vi "HFRR ADV v01.vi"() -> ()   [LabVIEW 2023] (continued)
        n1660 = property on="Language Selection" class="Enum (strict)"("Visible"=w1316) -> ()  [unwired: 2 in, 2 out]
        n1661 = property on="File Path" class="Path"("Disabled"=w1317) -> ()  [unwired: 2 in, 2 out]
        n1662 = property on="TEMP INTERCEPT:" class="DigNum (strict)"("Disabled"=w1317) -> ()  [unwired: 2 in, 2 out]
        n1663 = property on="visa due" class="CmbBox"("Disabled"=w1317) -> ()  [unwired: 2 in, 2 out]
        n1664 = property on="AIR TEMP INTERCEPT:" class="DigNum (strict)"("Disabled"=w1317) -> ()  [unwired: 2 in, 2 out]
        n1665 = property on="CH-HUMIDITY DRY" class="DigNum (strict)"("Disabled"=w1317) -> ()  [unwired: 2 in, 2 out]
        n1666 = property on="CH-HUMIDITY WET" class="DigNum (strict)"("Disabled"=w1317) -> ()  [unwired: 2 in, 2 out]
        n1667 = property on="CH-POWER -" class="DigNum (strict)"("Disabled"=w1317) -> ()  [unwired: 2 in, 2 out]
        n1668 = property on="CH-HEATER" class="DigNum (strict)"("Disabled"=w1317) -> ()  [unwired: 2 in, 2 out]
        n1669 = property on="CH-POWER +" class="DigNum (strict)"("Disabled"=w1317) -> ()  [unwired: 2 in, 2 out]
        n1670 = property on="SrvM CP" class="Bool (strict)"("Disabled"=w1317) -> ()  [unwired: 2 in, 2 out]
        n1671 = property on="Stroke PID Gains" class="Clust (strict)"("Disabled"=w1317) -> ()  [unwired: 2 in, 2 out]
        n1672 = property on="STROKE GAIN :" class="DigNum (strict)"("Disabled"=w1317) -> ()  [unwired: 2 in, 2 out]
        n1673 = property on="LvdtOff" class="DigNum (strict)"("Disabled"=w1317) -> ()  [unwired: 2 in, 2 out]
        n1674 = property on="DISPLACEMENT :" class="DigNum (strict)"("Disabled"=w1317) -> ()  [unwired: 2 in, 2 out]
        n1675 = property on="Port 2 Error" class="Clust (strict)"("Visible"="EDIT") -> ()  [unwired: 2 in, 2 out]
        n1676 = property on="Port 1 Error" class="Clust (strict)"("Visible"="EDIT") -> ()  [unwired: 2 in, 2 out]
        n1677 = stacked-sequence {
          frame #0 {
            n1678 = local read "EDIT"() -> (w1368:bool)
            n1679 = case shown="False" w1368 {
              tunnel: [u8 2 ("Disabled") u8 0 ("Disabled")] -> _
              frame False {
                w1370 = FALSE
                n1680 = local write "Password"("") -> ()
                n1681 = property on="ENTER THE NEW PASSWORD" class="Str"("Visible"=w1370) -> ()  [unwired: 2 in, 2 out]
                n1682 = property on="ENTER CURRENT PASSWORD" class="Str"("Visible"=w1370) -> ()  [unwired: 2 in, 2 out]
                n1683 = property on="SrvM CP" class="Bool (strict)"("Visible"=w1370) -> ()  [unwired: 2 in, 2 out]
                n1684 = property on="Password" class="Str"("Visible"=w1370) -> ()  [unwired: 2 in, 2 out]
                n1685 = local write "x = y?"(w1370) -> ()
                n1686 = local write "SrvM CP"(w1370) -> ()
                n1687 = property on="message" class="Str"("Visible"=w1370) -> ()  [unwired: 2 in, 2 out]
              }
              frame True {
                w1373 = TRUE
                n1688 = property on="SrvM CP" class="Bool (strict)"("Visible"=w1373) -> ()  [unwired: 2 in, 2 out]
                n1689 = property on="Password" class="Str"("Visible"=w1373) -> ()  [unwired: 2 in, 2 out]
              }
            }
            "dipl pwd" <- "@143$\n" ("dipl pwd")
          }
          frame #1 {
            # "Gain password"
            n1690 = String To Byte Array(string="ENTER CURRENT PASSWORD") -> (unsigned byte array=w1378:u8[])
            n1691 = Search 1D Array(1D array=w1378, element=u8 10) -> (index of element=w1381:i32)  [unwired: 1 in]
            n1692 = Index Array(array=w1378, index=w1381) -> (element=w1377:u8)
            n1693 = Equal?(x=w1377, y=10) -> (x = y?=w1375:bool)
            n1694 = case shown="True" w1375 {
              frame False {
                n1695 = property on="ENTER THE NEW PASSWORD" class="Str"("Visible"=FALSE) -> ()  [unwired: 2 in, 2 out]
              }
              frame True {
                # "password"
                # "change password logic"
                n1696 = local read "dipl pwd"() -> (w1388:string)
                n1697 = local read "ENTER CURRENT PASSWORD"() -> (w1394:string)
                n1698 = String To Byte Array(string=w1394) -> (unsigned byte array=w1396:u8[])
                n1699 = Array Size(array=w1396) -> (size(s)=w1393:i32)
                n1700 = String To Byte Array(string=w1388) -> (unsigned byte array=w1389:u8[])
                n1701 = Array Size(array=w1389) -> (size(s)=w1391:i32)
                n1702 = for {
                  N: w1393 -> [_]
                  tunnel: w1396 -> [w1420]
                  tunnel: [w1418] -> w1397 mode=indexing
                  tunnel: w1393 -> [w1412]
                  i -> [w1413]
                  n1703 = Decrement(x=w1412) -> (x-1=w1410:i32)
                  n1704 = Index Array(array=w1420, index=w1413) -> (element=w1414:u8)
                  n1705 = Equal?(x=w1413, y=w1410) -> (x = y?=w1411:bool)
                  n1706 = Number To Decimal String(number=w1414) -> (decimal integer string=w1419:string)  [unwired: 1 in]
                  n1707 = Select(t="", s=w1411, f="\r") -> (s? t:f=w1416:string)
                  n1708 = Concatenate Strings(w1419, w1416) -> (w1418:string)
                }
                n1709 = for {
                  N: w1391 -> [_]
                  tunnel: w1389 -> [w1408]
                  tunnel: [w1406] -> w1390 mode=indexing
                  tunnel: w1391 -> [w1403]
                  i -> [w1404]
                  n1710 = Decrement(x=w1403) -> (x-1=w1402:i32)
                  n1711 = Index Array(array=w1408, index=w1404) -> (element=w1407:u8)
                  n1712 = Equal?(x=w1404, y=w1402) -> (x = y?=w1401:bool)
                  n1713 = Number To Decimal String(number=w1407) -> (decimal integer string=w1405:string)  [unwired: 1 in]
                  n1714 = Select(t="", s=w1401, f="\r") -> (s? t:f=w1398:string)
                  n1715 = Concatenate Strings(w1405, w1398) -> (w1406:string)
                }
                n1716 = local read "string"() -> (w1395:string)
                n1717 = Concatenate Strings(w1397) -> (w1385:string)
                n1718 = Concatenate Strings(w1390) -> (w1384:string)
                n1719 = Concatenate Strings(w1395) -> (w1392:string)
                n1720 = Equal?(x=w1385, y=w1384) -> (x = y?=w1383:bool)
                n1721 = Equal?(x=w1385, y=w1392) -> (x = y?=w1387:bool)
                n1722 = Or(x=w1387, y=w1383) -> (x .or. y?=w1386:bool)
                n1723 = case shown="True" w1386 {
                  frame False {
                  }
                  frame True {
                    n1724 = property on="ENTER THE NEW PASSWORD" class="Str"("Visible"=TRUE) -> ()  [unwired: 2 in, 2 out]
                  }
                }
              }
            }
          }
          frame #2 {
            n1725 = String To Byte Array(string="ENTER THE NEW PASSWORD") -> (unsigned byte array=w1423:u8[])
            n1726 = Search 1D Array(1D array=w1423, element=u8 10) -> (index of element=w1427:i32)  [unwired: 1 in]
            n1727 = Index Array(array=w1423, index=w1427) -> (element=w1425:u8)
            n1728 = Equal?(x=w1425, y=10) -> (x = y?=w1422:bool)
            n1729 = case shown="True" w1422 {
              frame False {
              }
              frame True {
                n1730 = local read "ENTER THE NEW PASSWORD"() -> (w1430:string)
                n1731 = String To Byte Array(string=w1430) -> (unsigned byte array=w1435:u8[])
                n1732 = Array Size(array=w1435) -> (size(s)=w1432:i32)
                n1733 = for {
                  N: w1432 -> [_]
                  tunnel: w1435 -> [w1448]
                  tunnel: [w1445] -> w1437 mode=indexing
                  tunnel: w1432 -> [w1440]
                  i -> [w1438]
                  n1734 = Index Array(array=w1448, index=w1438) -> (element=w1447:u8)
                  n1735 = Decrement(x=w1440) -> (x-1=w1441:i32)
                  n1736 = Equal?(x=w1438, y=w1441) -> (x = y?=w1442:bool)
                  n1737 = Number To Decimal String(number=w1447) -> (decimal integer string=w1446:string)  [unwired: 1 in]
                  n1738 = Select(t="", s=w1442, f="\r") -> (s? t:f=w1439:string)
                  n1739 = Concatenate Strings(w1446, w1439) -> (w1445:string)
                }
                n1740 = local write "SrvM CP"(FALSE) -> ()
                n1741 = local write "EDIT"(FALSE) -> ()
                n1742 = local read "file path"() -> (w1429:path)
                n1743 = Concatenate Strings(w1437) -> (w1431:string)
                n1744 = Delete(path (use dialog)=w1429) -> (deleted path=w1433:path)  [unwired: 4 in, 2 out]
                n1745 = call <vilib>:"Write Characters To File.vi"("append to file? (new file:F)"=FALSE, "character string"=w1431, "file path (dialog if empty)"=w1433) -> ()  [unwired: 2 in, 1 out]
              }
            }
          }
          frame #3 {
            n1746 = case shown="True" "SrvM CP" {
              frame False {
                w1451 = ""
                n1747 = property on="ENTER CURRENT PASSWORD" class="Str"("Visible"=FALSE) -> ()  [unwired: 2 in, 2 out]
                n1748 = local write "ENTER CURRENT PASSWORD"(w1451) -> ()
                n1749 = local write "ENTER THE NEW PASSWORD"(w1451) -> ()
              }
              frame True {
                n1750 = property on="ENTER THE NEW PASSWORD" class="Str"() -> ("Visible"=w1452:bool)  [unwired: 2 in, 2 out]
                n1751 = Not(x=w1452) -> (.not. x?=w1453:bool)
                n1752 = property on="ENTER CURRENT PASSWORD" class="Str"("Visible"=w1453) -> ()  [unwired: 2 in, 2 out]
              }
            }
          }
          frame #4 {
            n1753 = String To Byte Array(string="Password") -> (unsigned byte array=w1460:u8[])
            n1754 = Search 1D Array(1D array=w1460, element=u8 10) -> (index of element=w1458:i32)  [unwired: 1 in]
            n1755 = Index Array(array=w1460, index=w1458) -> (element=w1459:u8)
            n1756 = Equal?(x=w1459, y=10) -> (x = y?=w1455:bool)
            n1757 = case shown="True" w1455 {
              frame False {
              }
              frame True {
                # "password"
                # "password"
                n1758 = local read "Password"() -> (w1473:string)
                n1759 = String To Byte Array(string=w1473) -> (unsigned byte array=w1476:u8[])
                n1760 = Array Size(array=w1476) -> (size(s)=w1471:i32)
                n1761 = local read "file path"() -> (w1461:path)
                n1762 = for {
                  N: w1471 -> [_]
                  tunnel: w1476 -> [w1493]
                  tunnel: [w1491] -> w1477 mode=indexing
                  tunnel: w1471 -> [w1488]
                  i -> [w1489]
                  n1763 = Decrement(x=w1488) -> (x-1=w1487:i32)
                  n1764 = Index Array(array=w1493, index=w1489) -> (element=w1492:u8)
                  n1765 = Equal?(x=w1489, y=w1487) -> (x = y?=w1486:bool)
                  n1766 = Number To Decimal String(number=w1492) -> (decimal integer string=w1490:string)  [unwired: 1 in]
                  n1767 = Select(t="", s=w1486, f="\r") -> (s? t:f=w1483:string)
                  n1768 = Concatenate Strings(w1490, w1483) -> (w1491:string)
                }
                n1769 = String To Byte Array(string="@143$\n") -> (unsigned byte array=w1462:u8[])
                n1770 = Array Size(array=w1462) -> (size(s)=w1467:i32)
                n1771 = call <vilib>:"Read Characters From File.vi"("file path (dialog if empty)"=w1461) -> ("character string"=w1475:string)  [unwired: 5 in, 3 out]
                "string" <- w1475
                n1772 = for {
                  N: w1467 -> [_]
                  tunnel: w1462 -> [w1504]
                  tunnel: [w1502] -> w1465 mode=indexing
                  tunnel: w1467 -> [w1499]
                  i -> [w1500]
                  n1773 = Decrement(x=w1499) -> (x-1=w1498:i32)
                  n1774 = Index Array(array=w1504, index=w1500) -> (element=w1503:u8)
                  n1775 = Equal?(x=w1500, y=w1498) -> (x = y?=w1497:bool)
                  n1776 = Number To Decimal String(number=w1503) -> (decimal integer string=w1501:string)  [unwired: 1 in]
                  n1777 = Select(t="", s=w1497, f="\r") -> (s? t:f=w1494:string)
                  n1778 = Concatenate Strings(w1501, w1494) -> (w1502:string)
                }
                n1779 = Concatenate Strings(w1477) -> (w1469:string)
                n1780 = Concatenate Strings(w1475) -> (w1474:string)
                n1781 = Equal?(x=w1469, y=w1474) -> (x = y?=w1464:bool)
                n1782 = Concatenate Strings(w1465) -> (w1466:string)
                n1783 = Equal?(x=w1469, y=w1466) -> (x = y?=w1470:bool)
                n1784 = Or(x=w1464, y=w1470) -> (x .or. y?=w1463:bool)
                "x = y?" <- w1463
                n1785 = case shown="True" w1463 {
                  selector: w1463 -> [w1480 _]
                  tunnel: w1472 -> [_ _]
                  frame False {
                    n1786 = And(x=w1480, y=TRUE ("Visible")) -> (x .and. y?=w1481:bool)
                    n1787 = property on="message" class="Str"("Visible"=w1481) -> ()  [unwired: 2 in, 2 out]
                  }
                  frame True {
                    n1788 = property on="message" class="Str"("Visible"=FALSE) -> ()  [unwired: 2 in, 2 out]
                  }
                }
                n1789 = flat-sequence {
                  tunnel: [w1478] -> w1472
                  frame #0 {
                    w1478 = ""
                    n1790 = local write "Password"(w1478) -> ()
                  }
                }
              }
            }
          }
        }
        n1791 = case shown="True" "SrvM CP 2" {
          frame False {
          }
          frame True {
            n1792 = local read "FRIC. FORCE : 2"() -> (w1366:dbl)
            n1793 = local read "STROKE GAIN : 2"() -> (w1365:dbl)
            n1794 = local read "TEMPERATURE : 2"() -> (w1363:dbl)
            n1795 = local read "HUMIDITY: 2"() -> (w1361:dbl)
            n1796 = local read "DISPLACEMENT : 4"() -> (w1364:dbl)
            n1797 = local read "AIR TEMPERATURE : 2"() -> (w1362:dbl)
            n1798 = local read "TEMP INTERCEPT: 2"() -> (w1360:dbl)
            n1799 = local read "AIR TEMP INTERCEPT: 2"() -> (w1359:dbl)
            n1800 = local write "FRIC. FORCE :"(w1366) -> ()
            n1801 = local write "STROKE GAIN :"(w1365) -> ()
            n1802 = local write "TEMPERATURE :"(w1363) -> ()
            n1803 = local write "AIR TEMPERATURE :"(w1362) -> ()
            n1804 = local write "HUMIDITY:"(w1361) -> ()
            n1805 = local write "DISPLACEMENT :"(w1364) -> ()
            n1806 = local write "AIR TEMP INTERCEPT:"(w1360) -> ()
            n1807 = local write "TEMP INTERCEPT:"(w1359) -> ()
            n1808 = local write "SrvM CP 2"(FALSE ("SrvM CP 2")) -> ()
          }
        }
        n1809 = local read "STROKE GAIN : 2"() -> (w1335:dbl)
        n1810 = local read "FRIC. FORCE : 2"() -> (w1338:dbl)
        n1811 = local read "AIR TEMPERATURE : 2"() -> (w1326:dbl)
        n1812 = local read "DISPLACEMENT : 4"() -> (w1331:dbl)
        n1813 = local read "TEMPERATURE : 2"() -> (w1329:dbl)
        n1814 = local read "STROKE GAIN :"() -> (w1334:dbl)
        n1815 = local read "HUMIDITY: 2"() -> (w1322:dbl)
        n1816 = local read "FRIC. FORCE :"() -> (w1337:dbl)
        n1817 = local read "AIR TEMPERATURE :"() -> (w1325:dbl)
        n1818 = local read "DISPLACEMENT :"() -> (w1330:dbl)
        n1819 = local read "TEMPERATURE :"() -> (w1327:dbl)
        n1820 = local read "HUMIDITY:"() -> (w1321:dbl)
        n1821 = Subtract(x=w1322, y=w1321) -> (x-y=w1323:dbl)
        n1822 = Subtract(x=w1335, y=w1334) -> (x-y=w1333:dbl)
        n1823 = Subtract(x=w1338, y=w1337) -> (x-y=w1336:dbl)
        n1824 = Subtract(x=w1329, y=w1327) -> (x-y=w1328:dbl)
        n1825 = Subtract(x=w1331, y=w1330) -> (x-y=w1332:dbl)
        n1826 = Subtract(x=w1326, y=w1325) -> (x-y=w1324:dbl)
        n1827 = Divide(x=w1333, y=w1334) -> (x/y=w1353:dbl)
        n1828 = Divide(x=w1324, y=w1325) -> (x/y=w1348:dbl)
        n1829 = Divide(x=w1336, y=w1337) -> (x/y=w1356:dbl)
        n1830 = Divide(x=w1323, y=w1321) -> (x/y=w1345:dbl)
        n1831 = Divide(x=w1328, y=w1327) -> (x/y=w1349:dbl)
        n1832 = Divide(x=w1332, y=w1330) -> (x/y=w1352:dbl)
        n1833 = Multiply(x=w1353, y=100.0) -> (x*y=→"STROKE Calibration Error":dbl)
        n1834 = Multiply(x=w1348, y=100.0) -> (x*y=→"AIR TEMPERATURE  Calibration Error":dbl)
        n1835 = Multiply(x=w1356, y=100.0) -> (x*y=→"FRIC. FORCE Calibration Error":dbl)
        n1836 = Multiply(x=w1352, y=100.0) -> (x*y=→"DISPLACEMENT  Calibration Error":dbl)
        n1837 = Multiply(x=w1345, y=100.0) -> (x*y=→"HUMIDITY  Calibration Error":dbl)
        n1838 = Multiply(x=w1349, y=100.0) -> (x*y=→"TEMPERATURE  Calibration Error":dbl)
      }
    }
  }
  n1839 = while {
    tunnel: [w2809] -> _
    tunnel: [w2808] -> w42
    tunnel: w16 -> [_]
    i -> [w2809]
    stop <- w2808 stop-if-true
    n1840 = local read "Main Tab"() -> (w2792:T1)
    n1841 = local read "Main Tab"() -> (w2794:T1)
    n1842 = local read "EDIT"() -> (w2815:bool)
    n1843 = case shown="True" w2815 {
      tunnel: [FALSE TRUE] -> w2800
      frame False {
      }
      frame True {
      }
    }
    n1844 = case shown="\"About\"" w2792 {
      frame "Acquire" {
      }
      frame "Compare Files", Default {
      }
      frame "About" {
      }
    }
    n1845 = local read "Rate"() -> (w2814:dbl)
    n1846 = Divide(x=1.0, y=w2814) -> (x/y=w2810:dbl)
    "Time 2" <- w2810
    n1847 = property on="Time slide" class="Slide (strict)"("Scale.Range:Maximum"=2500.0) -> ()  [unwired: 2 in, 2 out]
    n1848 = local read "conststatus"() -> (w2796:dbl)
    n1849 = Equal?(x=w2794, y=T1."About" ("Main Tab")) -> (x = y?=w2806:bool)
    n1850 = property on="FF Calibration g" class="WFGraph (strict)"("Visible"=w2800) -> ()  [unwired: 2 in, 2 out]
    n1851 = property on="Lift" class="Bool (strict)"("Visible"=w2800) -> ()  [unwired: 2 in, 2 out]
    n1852 = property on="Threshold" class="DigNum (strict)"("Visible"=w2800) -> ()  [unwired: 2 in, 2 out]
    n1853 = property on="Time slide" class="Slide (strict)"("Visible"=w2800) -> ()  [unwired: 2 in, 2 out]
    n1854 = Select(t=u32 2500 ("milliseconds to wait"), s=w2806, f=u32 500 ("milliseconds to wait")) -> (s? t:f=w2804:u32)
    n1855 = Multiply(x=w2810, y=w2804) -> (x*y=w2812:dbl)
    n1856 = Wait (ms)(milliseconds to wait=u32 50) -> ()  [unwired: 1 out]
    n1857 = call "Elapsed Time2"("Time Target (s)"=w2812, "Auto Reset"=TRUE) -> ("Time has Elapsed"=w2801:bool)  [unwired: 10 in, 7 out]
    n1858 = Equal?(x=w2796, y=0.0) -> (x = y?=w2797:bool)
    n1859 = case shown="True" w2797 {
      frame False {
      }
      frame True {
        # "C:\\WinDucom\\calibrate WO 2391.dcf"
        n1860 = local write "Lan flag"(22) -> ()
        n1861 = local write "conststatus"(10.0 ("rpm value : 2")) -> ()
        n1862 = String To Path(string="C:\\LAB-IQ-NXT\\calibrate WO 2464.dcf") -> (path=w2821:path)
        n1863 = Open/Create/Replace File "Open File"(file path (use dialog)=w2821) -> (refnum out=w2819:refnum<file>)  [unwired: 5 in, 2 out]
        n1864 = for {
          N: 22 -> [_]
          tunnel: w2819 -> [w2830]
          i -> [w2824]
          (unwired) TRUE ("line mode (F)")
          n1865 = Read from Text File "Read File"(file (use dialog)=w2830) -> (text=w2829:string)  [unwired: 3 in, 3 out]
          n1866 = Match Pattern(string=w2829, regular expression="]") -> (after substring=w2827:string)  [unwired: 1 in, 3 out]
          n1867 = String Subset(string=w2829, offset (0)=5, length (rest)=10 ("length (rest)")) -> (substring=w2822:string)
          n1868 = Fract/Exp String To Number(string=w2822) -> (number=w2823:dbl)  [unwired: 3 in, 1 out]
          n1869 = Match Pattern(string=w2827, regular expression="-") -> (before substring=w2825:string)  [unwired: 1 in, 3 out]
          n1870 = case shown="0" w2824 {
            tunnel: w2823 -> [w2833 w2834 w2835 w2836 _ _ _ w2841 w2842 w2843 w2846 w2847 w2848 w2849 w2850 w2851 w2852 w2855 w2856 _ _ w2859 _]
            tunnel: w2825 -> [_ _ _ _ w2837 w2838 w2839 _ _ _ _ _ _ _ _ _ _ _ _ w2857 w2858 _ _]
            frame 0 {
              n1871 = local write "FRIC. FORCE :"(w2833) -> ()
            }
            frame 1 {
              n1872 = local write "TEMPERATURE :"(w2834) -> ()
            }
            frame 2 {
              n1873 = local write "HUMIDITY:"(w2835) -> ()
            }
            frame 3 {
              n1874 = local write "AIR TEMPERATURE :"(w2836) -> ()
            }
            frame 4 {
              n1875 = local write "Com Port 1"(w2837) -> ()
            }
            frame 5 {
              n1876 = local write "visa due"(w2838) -> ()
              n1877 = local write "Com Port 2"(w2838) -> ()
            }
            frame 6 {
              n1878 = String To Path(string=w2839) -> (path=w2840:path)
              n1879 = local write "File Path"(w2840) -> ()
              "String" <- w2839
            }
            frame 7 {
              n1880 = local write "DISPLACEMENT :"(w2841) -> ()
            }
            frame 8 {
              n1881 = local write "STROKE GAIN :"(w2842) -> ()
            }
            frame 9 {
              n1882 = local read "Stroke PID Gains"() -> (w2845:T9)
              n1883 = Bundle By Name(cluster=w2845, "Proportional Gain (Kc)"=w2843) -> (w2844:T9)
              n1884 = local write "Stroke PID Gains"(w2844) -> ()
            }
            frame 10 {
              n1885 = local write "Language Selection"(w2846) -> ()
            }
            frame 11 {
              n1886 = local write "CH-POWER +"(w2847) -> ()
            }
            frame 12 {
              n1887 = local write "CH-POWER -"(w2848) -> ()
            }
            frame 13 {
              n1888 = local write "CH-HEATER"(w2849) -> ()
            }
            frame 14 {
              n1889 = local write "CH-HUMIDITY WET"(w2850) -> ()
            }
            frame 15 {
              n1890 = local write "CH-HUMIDITY DRY"(w2851) -> ()
            }
            frame 16 {
              n1891 = local read "Stroke PID Gains"() -> (w2854:T9)
              n1892 = Bundle By Name(cluster=w2854, "Integral Time (Ti, min)"=w2852) -> (w2853:T9)
              n1893 = local write "Stroke PID Gains"(w2853) -> ()
            }
            frame 17 {
              n1894 = local write "AIR TEMP INTERCEPT:"(w2855) -> ()
            }
            frame 18 {
              n1895 = local write "TEMP INTERCEPT:"(w2856) -> ()
            }
            frame 19 {
              n1896 = local write "S.NO"(w2857) -> ()
            }
            frame 20 {
              n1897 = local write "Com Port 3"(w2858) -> ()
            }
            frame 21 {
              n1898 = local write "LvdtOff"(w2859) -> ()
            }
            frame 22, Default {
            }
          }
        }
      }
    }
    n1899 = case shown="True" w2801 {
      frame False {
        # "79.77669138"
        # "2.3554"
        n1900 = local read "FRIC. FORCE :"() -> (w2864:dbl)
        n1901 = local read "FF cal val"() -> (w2861:dbl[])
        n1902 = Multiply(x=w2864, y=79.77669138) -> (x*y=w2863:dbl)
        n1903 = Multiply(x=w2861, y=w2863) -> (x*y=→"FF Calibration g":dbl[])
        "Err Count" <- 0 ("y")
      }
      frame True {
        n1904 = stacked-sequence {
          frame #0 {
            n1905 = stacked-sequence {
              frame #0 {
                "Lift" <- TRUE ("Lift")
              }
            }
          }
          frame #1 {
            w2876 = 2500 ("y")
            n1906 = local read "FF1"() -> (w2871:dbl[])
            n1907 = local read "Ch1"() -> (w2867:dbl[])
            "Waveform Chart 2" <- w2867
            n1908 = Array Size(array=w2871) -> (size(s)=w2870:i32)
            n1909 = Insert Into Array(array=w2871, index=w2870, new element=w2867) -> (w2873:dbl[])
            n1910 = call-poly <vilib>:"Mean.vi"("X"=w2867) -> ("mean"=→"Raw Mean":dbl)  [unwired: 1 out]
            n1911 = local read "RUN"() -> (w2868:bool)
            n1912 = Array Size(array=w2873) -> (size(s)=w2877:i32)
            n1913 = case shown="False" w2868 {
              frame False {
                n1914 = local write "Frequency"(0.0 ("Frequency")) -> ()
              }
              frame True {
              }
            }
            n1915 = Subtract(x=w2877, y=w2876) -> (x-y=w2875:i32)
            n1916 = Greater?(x=w2877, y=w2876) -> (0:w2878:bool)
            n1917 = case shown="True" w2878 {
              tunnel: w2875 -> [_ w2882]
              tunnel: [w2880 w2884] -> w2869
              tunnel: w2873 -> [w2880 w2883]
              frame False {
              }
              frame True {
                n1918 = Delete From Array(array=w2883, length=w2882, index=0) -> (array with subset deleted=w2884:dbl[])  [unwired: 1 out]
                "Numeric" <- w2882
              }
            }
            "FF1" <- w2869
            "PID Ref" <- TRUE ("PID Ref")
          }
          frame #2 {
          }
          frame #3 {
            w2885 = 0.0 ("lower limit")
            w2917 = 0.0 ("lower limit")
            # "CONVERT TO N"
            # "DATA PROCESSING"
            # "115 mV/N"
            n1919 = local read "Fric Val"() -> (w2978:dbl[])
            n1920 = local read "FRIC. FORCE :"() -> (w2968:dbl)
            n1921 = local read "Air temp"() -> (w2969:dbl[])
            n1922 = local read "temp buf"() -> (w2972:dbl[])
            n1923 = call-poly <vilib>:"Mean.vi"("X"=w2969) -> ("mean"=w2909:dbl)  [unwired: 1 out]
            "Raw air temp" <- w2909
            n1924 = local read "humid"() -> (w2919:string)
            n1925 = Multiply(x=w2978, y=1.0) -> (x*y=w2979:dbl[])
            n1926 = Multiply(x=w2968, y=79.77669138) -> (x*y=w2966:dbl)
            n1927 = call-poly <vilib>:"Mean.vi"("X"=w2972) -> ("mean"=w2911:dbl)  [unwired: 1 out]
            "Raw specimen temp" <- w2911
            n1928 = case shown="0, Default" "Calibrating" {
              tunnel: w2911 -> [w3001 _]
              tunnel: [w3001 w3002] -> w2910
              tunnel: w2909 -> [_ w3002]
              frame 0, Default {
              }
              frame 1 {
              }
            }
            n1929 = local read "HUMIDITY:"() -> (w2982:dbl)
            n1930 = Multiply(x=w2979, y=w2966) -> (x*y=w2976:dbl[])
            n1931 = Add(x=w2909, y="Offset Air Temp") -> (x+y=w2904:dbl)
            n1932 = local read "AIR TEMPERATURE :"() -> (w2953:dbl)
            n1933 = Fract/Exp String To Number(string=w2919) -> (number=w2918:dbl)  [unwired: 3 in, 1 out]
            n1934 = local read "TEMPERATURE :"() -> (w2952:dbl)
            n1935 = call-poly <vilib>:"Mean.vi"("X"=w2976) -> ("mean"=w2977:dbl)  [unwired: 1 out]
            n1936 = Multiply(x=w2918, y=w2982) -> (x*y=w2974:dbl)
            n1937 = Subtract(x=w2976, y=w2977) -> (x-y=w2915:dbl[])
            n1938 = case shown="True" "Boolean 4" {
              tunnel: w2910 -> [_ w3008]
              tunnel: "Standard Temp. ( °c )" -> [_ w3007]
              frame False {
              }
              frame True {
                n1939 = local read "Captured Values"() -> (w3005:dbl[][])
                n1940 = local write "Boolean 4"(FALSE ("Boolean 4")) -> ()
                n1941 = Build Array(w3007, w3008) -> (w3006:dbl[])
                n1942 = Build Array (concatenate)(w3005, w3006) -> (w3003:dbl[][])
                n1943 = local write "Captured Values"(w3003) -> ()
              }
            }
            n1944 = local read "AIR TEMP INTERCEPT:"() -> (w2949:dbl)
            n1945 = Multiply(x=w2904, y=w2953) -> (x*y=w2906:dbl)
            n1946 = Absolute Value(x=w2915) -> (abs(x)=w2983:dbl[])
            n1947 = Multiply(x=w2911, y=w2952) -> (x*y=w2905:dbl)
            n1948 = In Range and Coerce(upper limit=100.0, x=w2974, lower limit=w2917) -> (coerced(x)=w2921:dbl)  [unwired: 1 out]
            n1949 = local read "TEMP INTERCEPT:"() -> (w2916:dbl)
            n1950 = local read "Humid Last buf"() -> (w2944:dbl[])
            n1951 = call-poly <vilib>:"RMS.vi"("X"=w2915) -> ("rms value"=w2914:dbl)  [unwired: 1 out]
            n1952 = call-poly <vilib>:"Mean.vi"("X"=w2983) -> ()  [unwired: 2 out]
            n1953 = local read "RUN"() -> (w2965:bool)
            n1954 = Add(x=w2906, y=w2949) -> (x+y=w2951:dbl)
            n1955 = Add(x=w2905, y=w2916) -> (x+y=w2950:dbl)
            n1956 = local read "FRICVALZ"() -> (w2989:dbl)
            n1957 = Replace Array Subset(array=w2944, new element=w2921, index=0) -> (w2940:dbl[])
            n1958 = call <vilib>:"Mean PtByPt.vi"("x"=w2950, "sample length"=10) -> ("mean"=w2970:dbl)  [unwired: 2 in, 1 out]
            "TEMP 2" <- w2970
            n1959 = Select(t=0.01 ("FF fil1"), s=w2965, f=0.1 ("FF fil1")) -> (s? t:f=w2961:dbl)
            n1960 = case shown="True" "FRICVALZ 2" {
              tunnel: w2914 -> [_ w3025]
              frame False {
              }
              frame True {
                n1961 = local write "FRICVALZ 2"(FALSE ("FRICVALZ")) -> ()
                "FRICVALZ" <- w3025
              }
            }
            n1962 = Subtract(x=w2914, y=w2989) -> (x-y=w2980:dbl)
            n1963 = local read "AIR TEMP"() -> (w2958:dbl)
            n1964 = Multiply(x=w2951, y=w2961) -> (x*y=w2962:dbl)
            n1965 = Subtract(x=w2921, y=w2917) -> (x-y=w2920:dbl)
            "Humidity" <- w2920
            n1966 = Rotate 1D Array(1:w2940, 2:1 ("n")) -> (0:w2941:dbl[])
            n1967 = Index Array(array=w2940, index #1=0 ("index"), index #2=3 ("index")) -> (element #1=w2929:dbl, element #2=w2928:dbl)
            n1968 = case shown="True" "Boolean 5" {
              frame False {
              }
              frame True {
                n1969 = local write "Captured Values"(dbl[][] [] ("Captured Values")) -> ()
                n1970 = local write "Boolean 5"(FALSE) -> ()
                n1971 = local write "Best Fit"(dbl[] [] ("Best Fit")) -> ()
              }
            }
            n1972 = local read "FF 2"() -> (w2991:dbl)
            n1973 = Subtract(x=1.0 ("y"), y=w2961) -> (x-y=w2959:dbl)
            n1974 = Divide(x=w2929, y=w2928) -> (x/y=w2936:dbl)
            n1975 = Multiply(x=w2959, y=w2958) -> (x*y=w2957:dbl)
            n1976 = Multiply(x=w2980, y=0.1 ("FF fil1")) -> (x*y=w2995:dbl)
            n1977 = local write "TEMP"(w2970) -> ()
            n1978 = Multiply(x=0.9 ("FF fil2"), y=w2991) -> (x*y=w2994:dbl)
            n1979 = local write "Humid Last buf"(w2941) -> ()
            n1980 = Add(x=w2962, y=w2957) -> (x+y=w2955:dbl)
            n1981 = local read "offfset corr"() -> (w2932:bool)
            n1982 = local read "ecr buf"() -> (w2902:dbl[])
            n1983 = Subtract(x=1.0, y=w2936) -> (x-y=w2935:dbl)
            n1984 = Add(x=w2995, y=w2994) -> (x+y=w2988:dbl)
            "FF 2" <- w2988
            n1985 = local read "NORMAL LOAD"() -> (w2975:dbl)
            n1986 = Not A Number/Path/Refnum?(number/path/refnum=w2955) -> (NaN/Path/Refnum?=w2956:bool)
            n1987 = Absolute Value(x=w2935) -> (abs(x)=w2934:dbl)
            n1988 = Not(x=w2932) -> (.not. x?=w2930:bool)
            n1989 = Select(t=0.0, s=w2956, f=w2955) -> (s? t:f=w2887:dbl)
            "AIR TEMP" <- w2887
            n1990 = Greater Or Equal?(x=w2934, y=0.05) -> (x >= y?=w2923:bool)
            n1991 = call-poly <vilib>:"Mean.vi"("X"=w2902) -> ("mean"=w2899:dbl)  [unwired: 1 out]
            n1992 = And(x=w2923, y=w2930) -> (x .and. y?=w2931:bool)
            n1993 = Not A Number/Path/Refnum?(number/path/refnum=w2920) -> (NaN/Path/Refnum?=w2981:bool)
            n1994 = case shown="True" w2981 {
              frame False {
              }
              frame True {
                n1995 = local write "Humidity"(0.0 ("Humidity 3")) -> ()
              }
            }
            n1996 = case shown="True" w2931 {
              tunnel: w2929 -> [_ w3019]
              tunnel: w2928 -> [_ w3018]
              frame False {
                w3013 = 5.0 ("y")
                n1997 = local read "cnter"() -> (w3015:dbl)
                n1998 = Increment(x=w3015) -> (x+1=w3012:dbl)
                n1999 = Greater Or Equal?(x=w3012, y=w3013) -> (x >= y?=w3014:bool)
                n2000 = Select(t=w3013, s=w3014, f=w3012) -> (s? t:f=w3011:dbl)
                n2001 = local write "cnter"(w3011) -> ()
              }
              frame True {
                n2002 = Subtract(x=w3019, y=w3018) -> (x-y=→"offset":dbl)
                "offfset corr" <- TRUE ("offfset corr")
                "cnter" <- 0.0 ("cnter")
              }
            }
            n2003 = Multiply(x=w2899, y="ECR_Gain") -> (x*y=w2898:dbl)
            n2004 = local read "TEMP"() -> (w2987:dbl)
            n2005 = local read "ecr"() -> (w2893:dbl)
            n2006 = Divide(x=w2988, y=w2975) -> (x/y=w2945:dbl)
            n2007 = local read "offfset corr"() -> (w2925:bool)
            n2008 = Multiply(x=w2898, y=0.2) -> (x*y=w2891:dbl)
            n2009 = Multiply(x=0.8, y=w2893) -> (x*y=w2892:dbl)
            n2010 = call "Elapsed Time11"("Time Target (s)"=1.0) -> ("Time has Elapsed"=w2889:bool)  [unwired: 11 in, 7 out]
            n2011 = local read "cnter"() -> (w2927:dbl)
            n2012 = Not A Number/Path/Refnum?(number/path/refnum=w2987) -> (NaN/Path/Refnum?=w2986:bool)
            n2013 = Not A Number/Path/Refnum?(number/path/refnum=w2988) -> (NaN/Path/Refnum?=w2985:bool)
            n2014 = Not A Number/Path/Refnum?(number/path/refnum=w2945) -> (NaN/Path/Refnum?=w2947:bool)
            n2015 = Add(x=w2891, y=w2892) -> (x+y=w2890:dbl)
            n2016 = Select(t=0.0, s=w2947, f=w2945) -> (s? t:f=→"COF 2":dbl)
            n2017 = case shown="True" w2889 {
              tunnel: w2887 -> [_ w2997]
              frame False {
              }
              frame True {
                "AirT" <- w2997
              }
            }
            n2018 = Equal?(x=5.0 ("y"), y=w2927) -> (x = y?=w2926:bool)
            n2019 = Compound Arithmetic op=OR(w2986, w2985) -> (w2984:bool)
            n2020 = Not A Number/Path/Refnum?(number/path/refnum=w2890) -> (NaN/Path/Refnum?=w2900:bool)
            n2021 = Compound Arithmetic op=AND(w2923, w2926, w2925) -> (w2922:bool)
            n2022 = case shown="True" w2984 {
              frame False {
              }
              frame True {
                n2023 = local write "TEMP"(0.0 ("TEMP")) -> ()
                n2024 = local write "reinit"(TRUE ("reinit")) -> ()
                n2025 = local write "FF 2"(0.0 ("FF 2")) -> ()
              }
            }
            n2026 = Select(t=0.0, s=w2900, f=w2890) -> (s? t:f=w2897:dbl)
            n2027 = case shown="True" w2922 {
              frame False {
              }
              frame True {
                n2028 = local write "offfset corr"(FALSE ("offfset corr")) -> ()
                n2029 = local write "offset"(0.0 ("offset")) -> ()
              }
            }
            n2030 = In Range and Coerce(upper limit=100.0, x=w2897, lower limit=w2885) -> ()  [unwired: 2 out]
            "ecr" <- w2885
          }
          frame #4 {
            n2031 = case shown="True" "Boolean 6" {
              frame False {
              }
              frame True {
                n2032 = local read "Captured Values"() -> (w3037:dbl[][])
                n2033 = Index Array(array=w3037, index (col) #1=0 ("disabled index (col)"), index (col) #2=1 ("index (col)")) -> (element #1=w3035:dbl[], element #2=w3033:dbl[])  [unwired: 2 in]
                n2034 = local write "Boolean 6"(FALSE ("Boolean 6")) -> ()
                n2035 = call <vilib>:"Linear Fit.vi"("Y"=w3035, "X"=w3033) -> ("Best Linear Fit"=→"Best Fit":dbl[], "slope"=w3029:dbl, "intercept"=w3028:dbl)  [unwired: 9 in, 2 out]
                "Slope" <- w3029
                "Intercept" <- w3028
                n2036 = local read "Calibrating"() -> (w3030:u16)
                n2037 = case shown="1" w3030 {
                  tunnel: w3029 -> [w3039 w3041]
                  tunnel: w3028 -> [w3038 w3040]
                  frame 0, Default {
                    n2038 = local write "TEMPERATURE :"(w3039) -> ()
                    n2039 = local write "TEMP INTERCEPT:"(w3038) -> ()
                  }
                  frame 1 {
                    n2040 = local write "AIR TEMPERATURE :"(w3041) -> ()
                    n2041 = local write "AIR TEMP INTERCEPT:"(w3040) -> ()
                  }
                }
              }
            }
            n2042 = flat-sequence {
              frame #0 {
                n2043 = Wait (ms)(milliseconds to wait=u32 100) -> ()  [unwired: 1 out]
              }
              frame #1 {
                n2044 = local write "Lift"(FALSE ("Lift")) -> ()
              }
            }
          }
        }
      }
    }
    n2045 = local read "EXIT"() -> (w2808:bool)
    "Rate" <- 2500.0 ("No of Samples")
    "Humid Last buf" <- dbl[] [0.0, 0.0, 0.0, 0.0] ("Humid Last buf")
  }
  n2046 = VISA Close(VISA resource name=w12, error in (no error)=w11) -> (error out=w13:errorcluster)
  n2047 = call <vilib>:"Clear Errors.vi"("error in (no error)"=w13) -> ()  [unwired: 5 in, 2 out]
  n2048 = VISA Close(VISA resource name=w40, error in (no error)=w39) -> (error out=w37:errorcluster)
  n2049 = call <vilib>:"Clear Errors.vi"("error in (no error)"=w37) -> ()  [unwired: 5 in, 2 out]
  n2050 = Or(x=w27, y=w26) -> (x .or. y?=w28:bool)
  n2051 = while {
    tunnel: [w3103] -> w33
    shift-right: [w3083] -> _
    shift-left: "" -> [w3071]
    tunnel: [w3059] -> _
    i -> [w3059]
    stop <- w3103 stop-if-true
    w3085 = ";" ("string")
    n2052 = local read "start en"() -> (w3105:bool)
    n2053 = And(x="st enable", y=w3105) -> (x .and. y?=w3106:bool)
    n2054 = local read "ACQUIRE 3"() -> (w3048:bool)
    n2055 = local read "Elapsed time"() -> (w3067:dbl)
    n2056 = case shown="True" w3106 {
      tunnel: "st enable" -> [w3170 w3171]
      tunnel: [w3170 w3171] -> w3049
      frame False {
      }
      frame True {
        n2057 = local write "start en"(FALSE ("start en")) -> ()
      }
    }
    n2058 = Wait (ms)(milliseconds to wait=u32 80) -> ()  [unwired: 1 out]
    n2059 = local read "Stroke"() -> (w3058:dbl)
    n2060 = Greater?(x=w3067, y=0.1) -> (0:w3065:bool)
    n2061 = Or(x=w3049, y=w3048) -> (x .or. y?=w3050:bool)
    n2062 = case shown="True" "ACQUIRE 2" {
      frame False {
      }
      frame True {
        n2063 = call "Elapsed Time13"() -> ("Time has Elapsed"=w3113:bool)  [unwired: 12 in, 7 out]
        n2064 = case shown="True" w3113 {
          frame False {
          }
          frame True {
            n2065 = local write "ACQUIRE 2"(FALSE ("ACQUIRE 2")) -> ()
            n2066 = local write "ACQUIRE 3"(FALSE ("ACQUIRE 2")) -> ()
          }
        }
        n2067 = local write "ACQUIRE 3"(TRUE ("ACQUIRE 2")) -> ()
      }
    }
    n2068 = case shown="True" w3050 {
      tunnel: w3058 -> [_ w3193]
      tunnel: [w3173 _] -> w3102
      tunnel: w3065 -> [_ _]
      tunnel: w3048 -> [_ w3180]
      frame False {
        w3173 = TRUE ("PID Rst")
        n2069 = local read "stop cmd"() -> (w3174:bool)
        n2070 = case shown="True" w3174 {
          frame False {
          }
          frame True {
            n2071 = local write "stop cmd"(FALSE ("stop cmd")) -> ()
          }
        }
        n2072 = local write "PID Rst"(TRUE ("PID Rst")) -> ()
        "start en" <- w3173
      }
      frame True {
        w3200 = cluster{"output high":dbl, "output low":dbl} {"output high"=600.0, "output low"=-600.0} ("output range")
        n2073 = local read "STROKE GAIN :"() -> (w3185:dbl)
        n2074 = call "Elapsed Time6"("Reset"="PID Rst", "Auto Reset"=FALSE) -> ("Time has Elapsed"=w3194:bool)  [unwired: 10 in, 7 out]
        n2075 = Multiply(x="Set Strk", y=w3185) -> (x*y=w3178:dbl)
        n2076 = case shown="False" w3194 {
          tunnel: [w3205 w3206] -> w3197
          tunnel: "Set Strk" -> [w3205 _]
          tunnel: w3193 -> [_ w3206]
          frame False {
          }
          frame True {
          }
        }
        n2077 = Multiply(x=w3178, y=1.0) -> (x*y=w3177:dbl)
        n2078 = Select(t=T9 {"Proportional Gain (Kc)"=0.0, "Integral Time (Ti, min)"=0.02, "Derivative Time (Td, min)"=0.0} ("Stroke PID Gains"), s=w3180, f="Stroke PID Gains") -> (s? t:f=w3181:T9)
        n2079 = Not(x=w3194) -> (.not. x?=w3192:bool)
        n2080 = call-poly <vilib>:"PID.vi"("reinitialize? (F)"=w3192, "output range"=w3200, "PID gains"=w3181, "process variable"=w3197, "setpoint"="Set Strk") -> ("output"=w3191:dbl)  [unwired: 5 in, 1 out]
        "Slide 5" <- w3191
        n2081 = Select(t=w3191, s=w3194, f=0.0) -> (s? t:f=w3195:dbl)
        n2082 = flat-sequence {
          tunnel: w3195 -> [_]
          frame #0 {
            n2083 = local write "PID Rst"(FALSE ("PID Rst")) -> ()
          }
        }
        n2084 = Add(x=w3177, y=w3195) -> (x+y=w3190:dbl)
        n2085 = Unbundle(w3200) -> ("output high"=w3199:dbl, "output low"=w3198:dbl)
        n2086 = To Word Integer(number=w3190) -> (16bit integer=w3187:i16)
        n2087 = property on="Slide 5" class="Slide (strict)"("Scale.Range:Minimum"=w3198, "Scale.Range:Maximum"=w3199) -> ()  [unwired: 2 in, 2 out]
        n2088 = In Range and Coerce(upper limit=4095.0 ("f"), x=w3187, lower limit=100.0 ("f")) -> (coerced(x)=w3184:dbl)  [unwired: 1 out]
        "PID Out" <- w3184
        n2089 = Number To Decimal String(number=w3184) -> (decimal integer string=→"st gain":string)  [unwired: 1 in]
        "stop cmd" <- TRUE ("Auto Reset")
      }
    }
    n2090 = flat-sequence {
      frame #0 {
        n2091 = local read "CH-POWER +"() -> (w3117:u16)
        n2092 = local read "CH-POWER -"() -> (w3118:u16)
        n2093 = case shown="1" w3118 {
          tunnel: "PWR" -> [w3119 w3120 w3121 w3122 w3123 w3124 w3125 w3126]
          frame 0, Default {
            n2094 = local write "Do 0"(w3119) -> ()
          }
          frame 1 {
            n2095 = local write "Do 1"(w3120) -> ()
          }
          frame 2 {
            n2096 = local write "Do 2"(w3121) -> ()
          }
          frame 3 {
            n2097 = local write "Do 3"(w3122) -> ()
          }
          frame 4 {
            n2098 = local write "Do 4"(w3123) -> ()
          }
          frame 5 {
            n2099 = local write "Do 5"(w3124) -> ()
          }
          frame 6 {
            n2100 = local write "Do 6"(w3125) -> ()
          }
          frame 7 {
            n2101 = local write "Do 7"(w3126) -> ()
          }
        }
        n2102 = case shown="1" w3117 {
          tunnel: "PWR" -> [w3127 w3128 w3129 w3130 w3131 w3132 w3133 w3134]
          frame 0, Default {
            n2103 = local write "Do 0"(w3127) -> ()
          }
          frame 1 {
            n2104 = local write "Do 1"(w3128) -> ()
          }
          frame 2 {
            n2105 = local write "Do 2"(w3129) -> ()
          }
          frame 3 {
            n2106 = local write "Do 3"(w3130) -> ()
          }
          frame 4 {
            n2107 = local write "Do 4"(w3131) -> ()
          }
          frame 5 {
            n2108 = local write "Do 5"(w3132) -> ()
          }
          frame 6 {
            n2109 = local write "Do 6"(w3133) -> ()
          }
          frame 7 {
            n2110 = local write "Do 7"(w3134) -> ()
          }
        }
      }
    }
    n2111 = local read "RUN"() -> (w3056:bool)
    n2112 = Or(x=w3056, y="ACQUIRE 3") -> (x .or. y?=w3055:bool)
    n2113 = local read "Set Hz"() -> (w3073:dbl)
    n2114 = Select(t=w3073, s=w3055, f=0.0) -> (s? t:f=w3072:dbl)
    n2115 = local read "st gain"() -> (w3076:string)
    n2116 = local read "DO"() -> (w3077:string)
    n2117 = case shown="True" "Boolean 10" {
      frame False {
      }
      frame True {
        n2118 = local write "Tab Control 8"(enum32{"setup", "calibrate"}."calibrate" ("Tab Control 8")) -> ()
        n2119 = local write "Boolean 10"(FALSE ("Boolean 10")) -> ()
      }
    }
    n2120 = Number To Decimal String(number=w3072) -> (decimal integer string=w3075:string)  [unwired: 1 in]
    n2121 = case shown="True" "Boolean 11" {
      frame False {
      }
      frame True {
        n2122 = local write "Tab Control 8"(enum32{"setup", "calibrate"}."setup" ("Tab Control 8")) -> ()
        n2123 = local write "Boolean 11"(FALSE ("Boolean 11")) -> ()
      }
    }
    n2124 = String Length(string=w3076) -> (length=w3091:i32)
    n2125 = String Length(string=w3077) -> (length=w3079:i32)
    n2126 = String Length(string=w3075) -> (length=w3092:i32)
    n2127 = Subtract(x=4.0, y=w3091) -> (x-y=w3088:dbl)
    n2128 = Subtract(x=3.0, y=w3079) -> (x-y=w3082:dbl)
    n2129 = flat-sequence {
      tunnel: w3102 -> [_]
      frame #0 {
        n2130 = Build Array("Do 0", "Do 1", "Do 2", "Do 3", "Do 4", "Do 5", "Do 6", "Do 7") -> (w3161:bool[])
        n2131 = Boolean Array To Number(Boolean array=w3161) -> (number=w3159:u32)
        n2132 = Add(x=w3159, y=u32 0) -> (x+y=w3157:u32)
        n2133 = Number To Decimal String(number=w3157) -> (decimal integer string=→"DO":string)  [unwired: 1 in]
      }
    }
    n2134 = Subtract(x=3.0, y=w3092) -> (x-y=w3093:dbl)
    n2135 = Replace Substring(3:w3088, 4:w3076, 5:"0000" ("string")) -> (1:w3086:string)  [unwired: 1 in, 1 out]
    n2136 = Replace Substring(3:w3082, 4:w3077, 5:"000" ("string")) -> (1:w3078:string)  [unwired: 1 in, 1 out]
    n2137 = Replace Substring(3:w3093, 4:w3075, 5:"000" ("string")) -> (1:w3087:string)  [unwired: 1 in, 1 out]
    n2138 = Concatenate Strings("*" ("string"), w3087, w3085, w3086, w3085, w3078, "$" ("string")) -> (w3083:string)
    "Stroke_send_Val" <- w3083
    n2139 = local read "RUN"() -> (w3053:bool)
    n2140 = local read "ACQUIRE 3"() -> (w3052:bool)
    n2141 = local read "send"() -> (w3069:bool)
    n2142 = Not Equal?(x=w3071, y=w3083) -> (x != y?=w3084:bool)
    n2143 = Or(x=w3053, y=w3052) -> (x .or. y?=w3051:bool)
    n2144 = And(x=w3069, y=w3051) -> (x .and. y?=w3068:bool)
    n2145 = Or(x=w3084, y=w3068) -> (x .or. y?=w3062:bool)
    n2146 = case shown="False" w3051 {
      frame False {
        "send" <- TRUE ("send")
      }
      frame True {
      }
    }
    n2147 = call "Elapsed Time4"("Time Target (s)"=0.5) -> ("Time has Elapsed"=w3060:bool)  [unwired: 11 in, 7 out]
    n2148 = local read "Din"() -> (w3101:u8[])
    n2149 = Or(x=w3060, y=w3062) -> (x .or. y?=w3061:bool)
    n2150 = Index Array(array=w3101, index=0) -> (element=w3099:u8)
    n2151 = case shown="True" w3061 {
      tunnel: w3083 -> [_ w3138]
      frame False {
      }
      frame True {
        n2152 = local read "Due Com"() -> (w3139:string[])
        n2153 = Build Array (concatenate)(w3139, w3138) -> (→"Due Com":string[])
        n2154 = local write "send"(FALSE ("send")) -> ()
      }
    }
    n2155 = Number To Boolean Array(number=w3099) -> (Boolean array=w3098:bool[])
    n2156 = Array Size(array=w3098) -> (size(s)=w3097:i32)
    n2157 = Greater Than 0?(x=w3097) -> (x > 0?=w3096:bool)
    n2158 = case shown="True" w3096 {
      tunnel: w3098 -> [_ w3153]
      frame False {
      }
      frame True {
        n2159 = Index Array(array=w3153, index #1=0 ("index"), index #2=1 ("index"), index #3=2 ("index"), index #4=3 ("index"), index #5=4 ("index"), index #6=5 ("index"), index #7=6 ("index"), index #8=7 ("index")) -> (element #1=→"DI 0":bool, element #2=→"DI 1":bool, element #3=→"DI 2":bool, element #4=→"DI 3":bool, element #5=→"DI 4":bool, element #6=→"DI 5":bool, element #7=→"DI 6":bool, element #8=→"DI 7":bool)
      }
    }
    n2160 = local read "EXIT"() -> (w3103:bool)
  }
  n2161 = Or(x=w18, y=w28) -> (x .or. y?=w35:bool)
  n2162 = control-ref of="new picture"() -> ()  [unwired: 1 out]
  n2163 = while {
    tunnel: w16 -> [_]
    tunnel: [w3209] -> w46
    tunnel: [w3208] -> _
    i -> [w3208]
    stop <- w3209 stop-if-true
    n2164 = local read "PID-out"() -> (w3210:dbl)
    "Slide 2" <- w3210
    n2165 = Greater Or Equal?(x=w3210, y=2.0) -> (x >= y?=w3211:bool)
    n2166 = flat-sequence {
      tunnel: w3211 -> [w3219]
      tunnel: w3210 -> [w3222]
      tunnel: [w3220] -> w3217
      tunnel: [w3218] -> w3216
      tunnel: [w3238] -> w3215
      tunnel: w3217 -> [w3238]
      tunnel: w3216 -> [w3235]
      tunnel: [w3235] -> w3214
      tunnel: w3215 -> [w3240]
      tunnel: [w3239] -> w3213
      tunnel: w3214 -> [w3239]
      tunnel: w3213 -> [w3254]
      frame #0 {
        n2167 = case shown="True" w3219 {
          selector: w3219 -> [w3224 _]
          frame False {
            n2168 = local write "HEATER"(w3224) -> ()
          }
          frame True {
            w3226 = TRUE ("data")
            n2169 = local read "CH-HEATER"() -> (w3225:u16)
            n2170 = case shown="2" w3225 {
              tunnel: w3226 -> [w3227 w3228 w3229 w3230 w3231 w3232 w3233 w3234]
              frame 0, Default {
                n2171 = local write "Do 0"(w3227) -> ()
              }
              frame 1 {
                n2172 = local write "Do 1"(w3228) -> ()
              }
              frame 2 {
                n2173 = local write "Do 2"(w3229) -> ()
              }
              frame 3 {
                n2174 = local write "Do 3"(w3230) -> ()
              }
              frame 4 {
                n2175 = local write "Do 4"(w3231) -> ()
              }
              frame 5 {
                n2176 = local write "Do 5"(w3232) -> ()
              }
              frame 6 {
                n2177 = local write "Do 6"(w3233) -> ()
              }
              frame 7 {
                n2178 = local write "Do 7"(w3234) -> ()
              }
            }
            "HEATER" <- w3226
          }
        }
        n2179 = Select(t=w3222, s=w3219, f=0.0) -> (s? t:f=w3218:dbl)
        n2180 = Greater Or Equal?(x=w3222, y=97.0) -> (x >= y?=w3220:bool)
      }
      frame #1 {
        n2181 = Multiply(x=w3235, y=5.0) -> (x*y=w3237:dbl)
        n2182 = Wait (ms)(milliseconds to wait=w3237) -> ()  [unwired: 1 out]
      }
      frame #2 {
        n2183 = case shown="True" w3240 {
          frame False {
            w3241 = FALSE ("data")
            n2184 = local write "HEATER"(w3241) -> ()
            n2185 = local read "CH-HEATER"() -> (w3242:u16)
            n2186 = case shown="4" w3242 {
              tunnel: w3241 -> [w3243 w3244 w3245 w3246 w3247 w3248 w3249 w3250]
              frame 0, Default {
                n2187 = local write "Do 0"(w3243) -> ()
              }
              frame 1 {
                n2188 = local write "Do 1"(w3244) -> ()
              }
              frame 2 {
                n2189 = local write "Do 2"(w3245) -> ()
              }
              frame 3 {
                n2190 = local write "Do 3"(w3246) -> ()
              }
              frame 4 {
                n2191 = local write "Do 4"(w3247) -> ()
              }
              frame 5 {
                n2192 = local write "Do 5"(w3248) -> ()
              }
              frame 6 {
                n2193 = local write "Do 6"(w3249) -> ()
              }
              frame 7 {
                n2194 = local write "Do 7"(w3250) -> ()
              }
            }
          }
          frame True {
          }
        }
      }
      frame #3 {
        n2195 = Subtract(x=100, y=w3254) -> (x-y=w3253:dbl)
        n2196 = Multiply(x=w3253, y=5.0) -> (x*y=w3251:dbl)
        n2197 = Wait (ms)(milliseconds to wait=w3251) -> ()  [unwired: 1 out]
      }
    }
    n2198 = local read "EXIT"() -> (w3209:bool)
  }
  n2199 = Or(x=w42, y=w35) -> (x .or. y?=w32:bool)
  n2200 = Or(x=w32, y=w33) -> (x .or. y?=w21:bool)
  n2201 = while {
    shift-right: [w3297] -> w9
    shift-left: errorcluster {"status"=TRUE, "code"=0, "source"="Init"} ("error out") -> [w3261]
    shift-right: [w3296] -> w8
    shift-left: _ -> [w3262]
    shift-right: [w3295] -> _
    shift-left: "" -> [w3294]
    tunnel: [w3293] -> w22
    shift-right: ["Set Rh"] -> _
    shift-left: 0.0 ("Set Rh") -> [w3287]
    tunnel: [w3264] -> _
    i -> [w3264]
    stop <- w3293 stop-if-true
    n2202 = local read "Com Port 3"() -> (w3263:refnum<visa-resource-name>)
    n2203 = flat-sequence {
      tunnel: w3261 -> [w3300]
      tunnel: [w3300] -> w3260
      frame #0 {
        n2204 = Wait (ms)(milliseconds to wait=u32 200) -> ()  [unwired: 1 out]
      }
    }
    n2205 = Not Equal?(x=w3263, y=w3262) -> (x != y?=w3258:bool)
    n2206 = Or(x=w3258, y="Re-Initialise") -> (x .or. y?=w3257:bool)
    n2207 = case shown="True" w3257 {
      tunnel: w3260 -> [w3298 _]
      tunnel: [w3298 errorcluster {"status"=TRUE, "code"=0, "source"="Init"} ("error out")] -> w3259
      frame False {
      }
      frame True {
      }
    }
    n2208 = case shown="No Error" w3259 {
      selector: w3259 -> [w3325 w3371]
      tunnel: [w3323 w3364] -> w3297
      tunnel: w3262 -> [w3326 w3370]
      tunnel: [w3324 w3373] -> w3296
      tunnel: w3294 -> [w3313 w3372]
      tunnel: [w3320 w3372] -> w3295
      frame No Error {
        n2209 = call "Elapsed Time7"() -> ("Time has Elapsed"=w3319:bool)  [unwired: 12 in, 7 out]
        n2210 = Not Equal?(x="Humidity Str Send", y=w3313) -> (x != y?=w3315:bool)
        n2211 = Or(x=w3315, y=w3319) -> (x .or. y?=w3318:bool)
        n2212 = Select(t="Humidity Str Send", s=w3315, f="vals" ("regular expression")) -> (s? t:f=w3314:string)
        n2213 = Or(x=w3318, y="Send") -> (x .or. y?=w3322:bool)
        n2214 = case shown="True" w3322 {
          tunnel: [w3329 w3334] -> w3323
          tunnel: w3326 -> [w3328 w3342]
          tunnel: w3325 -> [w3329 w3341]
          tunnel: [w3328 w3335] -> w3324
          tunnel: w3314 -> [_ w3340]
          tunnel: [w3327 w3331] -> w3320
          tunnel: "Humidity Str Send" -> [_ w3332]
          tunnel: w3315 -> [_ w3333]
          tunnel: w3313 -> [w3327 w3330]
          frame False {
          }
          frame True {
            n2215 = flat-sequence {
              tunnel: w3342 -> [w3350]
              tunnel: w3341 -> [w3349]
              tunnel: w3340 -> [w3346]
              tunnel: [w3348] -> w3339
              tunnel: [w3347] -> w3338
              tunnel: w3339 -> [w3353]
              tunnel: w3338 -> [w3352]
              tunnel: [w3353] -> w3337
              tunnel: [w3352] -> w3336
              tunnel: w3337 -> [w3360]
              tunnel: w3336 -> [w3359]
              tunnel: [w3358] -> w3335
              tunnel: [w3357] -> w3334
              frame #0 {
                n2216 = Concatenate Strings(w3346, "\r") -> (w3345:string)
                n2217 = local write "Ser Led"(TRUE ("Boolean 4")) -> ()
